vi "Parse Config Header.vi"(8 "error in (no error)":errorcluster, 10 "Config String":string) -> (0 "error out":errorcluster, 1 "type":string, 2 "file":string, 3 "name":string)   [LabVIEW 2020, in "JMETestSolutions.Instrument.lvlib" / "JMETestSolutions.Instrument.lvclass"]
uses:
  JMETestSolutions.Instrument.lvclass
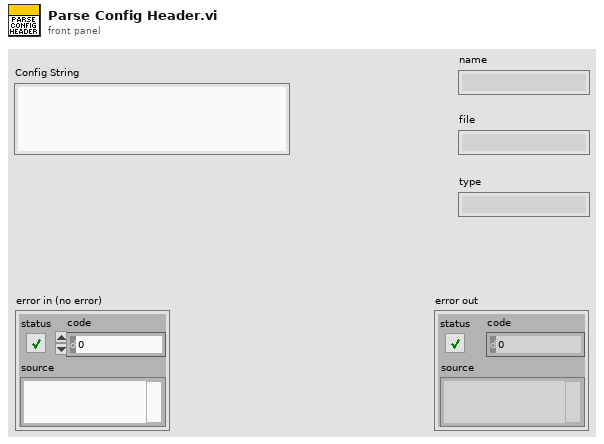
[diagram p1: front panel]
types:
  T1 = cluster{"name":string, "file":string, "type":string}
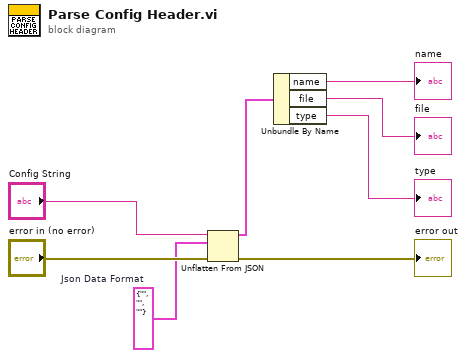
[diagram p0: block diagram]
diagram:
  w5 = T1 {"name"="", "file"="", "type"=""}  # Json Data Format
  n1 = Unflatten From JSON(JSON string="Config String", type and defaults=w5, error in (no error)="error in (no error)") -> (value=w4:T1, error out=→"error out":errorcluster)  [unwired: 4 in]
  n2 = Unbundle By Name(w4) -> ("name"=→"name":string, "file"=→"file":string, "type"=→"type":string)
